vi "SpotFinder.vi"(0 "first scan?":bool, 1 "auto":bool, 4 "Int duplex?":refnum<vi>, 5 "notes":refnum<vi>, 6 "router 3":refnum<vi>, 7 "plane 2":refnum<vi>, 8 "Image Path":refnum<vi>, 9 "16bit?":refnum<vi>, 10 "TACwinLoaded?":refnum<vi>) -> ()   [LabVIEW 2009]
panel:
  out "already x spots":i16
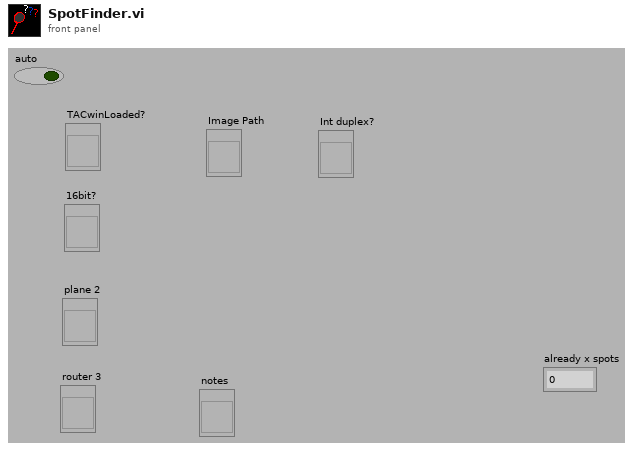
[diagram p1: front panel]
types:
  T1 = enum16{"Ini", "Dump", "Colorpal", "Input", "Get"}
  T2 = enum16{"Display", "change", "get", "save", "create text", "load", "Get Refnum"}
  T3 = enum16{"Ini", "Get", "Set", "Refresh", "dump", "move", "name"}
  T4 = typedef "spotproperties.ctl" = cluster{"draw?":bool, "plane":u32, "Coordinates":i32[], "TACWindow":cluster{"TACWindow1":i32, "TACWindow2":i32}, "Lifetime[ns]":ext[], "tauerror":dbl[], "F2-Value overall":dbl, "overall intensity":u32[], "F2-Value TAC":dbl, "TAC intensity":u32[], "Decay":u32[][]}
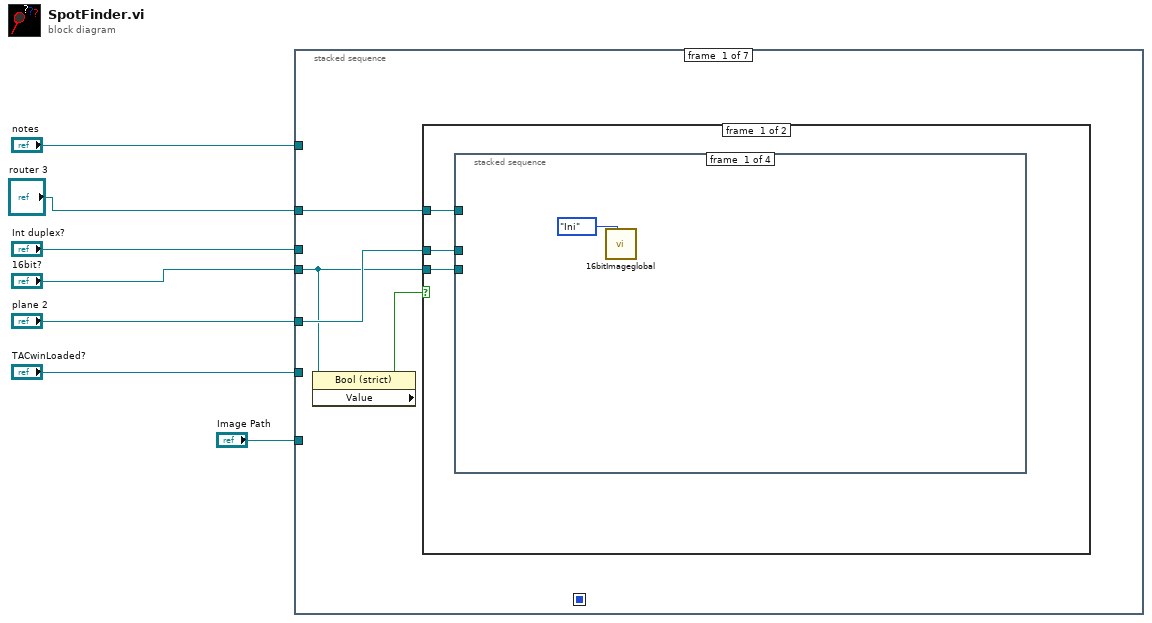
[diagram p0: block diagram]
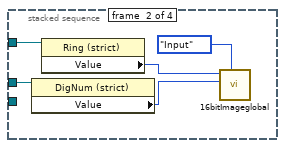
[diagram p2: hidden frame]
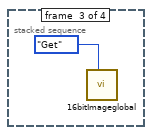
[diagram p3: hidden frame]
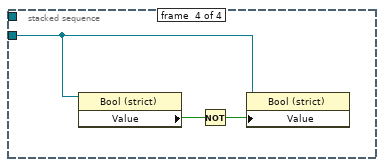
[diagram p4: hidden frame]
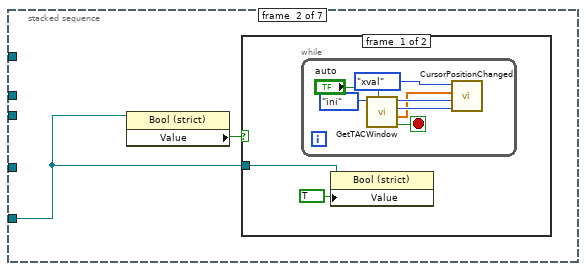
[diagram p6: hidden frame]
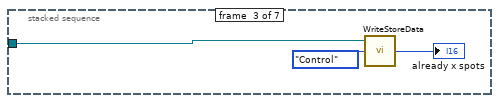
[diagram p8: hidden frame]
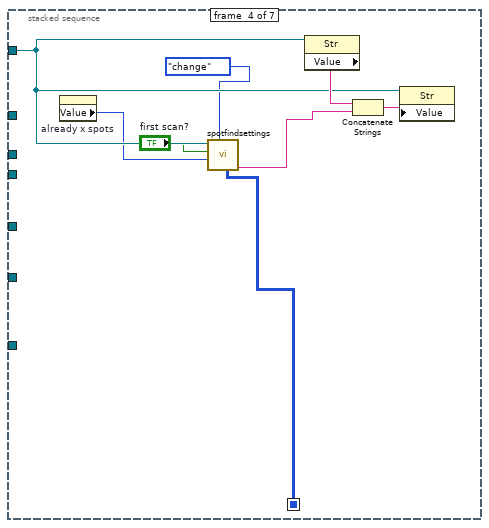
[diagram p9: hidden frame]
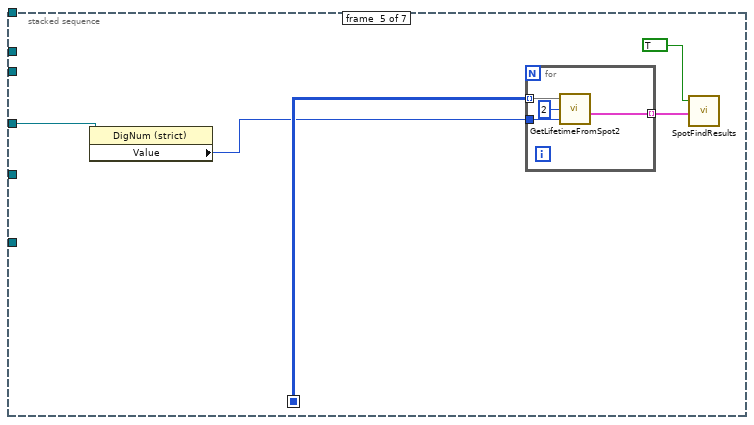
[diagram p10: hidden frame]
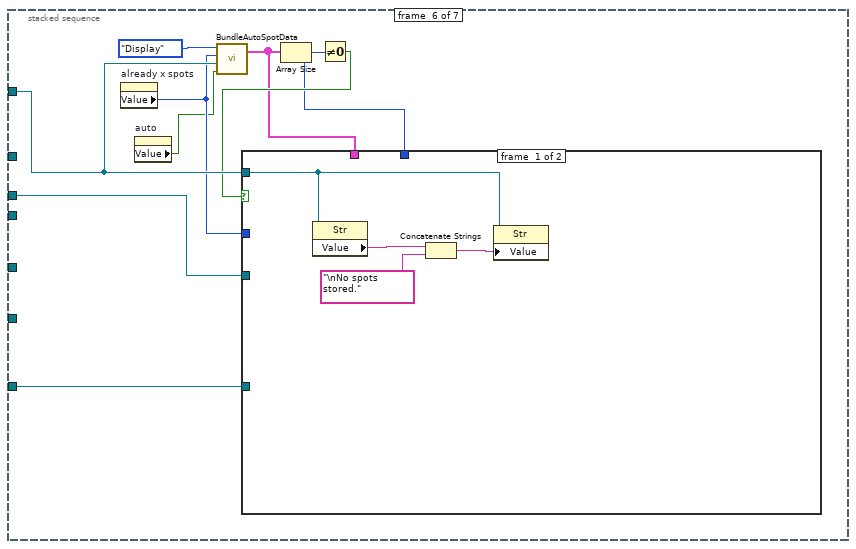
[diagram p11: hidden frame]
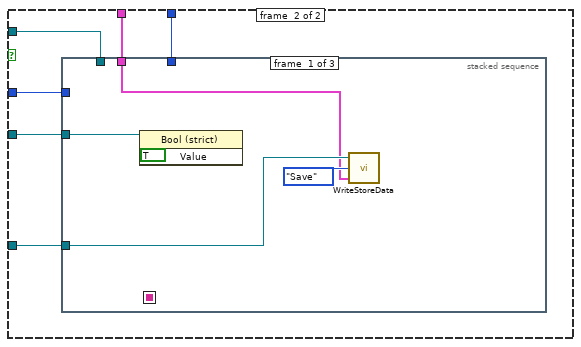
[diagram p12: hidden frame]
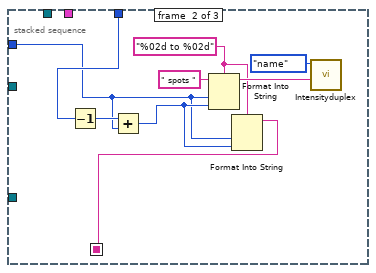
[diagram p13: hidden frame]
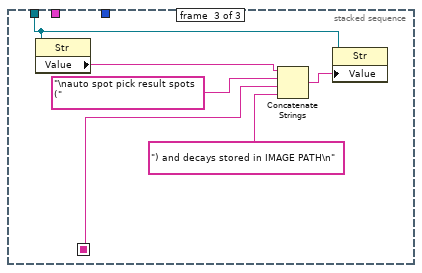
[diagram p14: hidden frame]
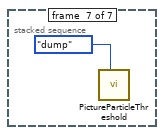
[diagram p15: hidden frame]
diagram:
  n1 = stacked-sequence {
    seq-local: [_ _ _ w40 _ _ _] -> [_ _ _ _ w51 _ _]
    tunnel: "TACwinLoaded?" -> [_ w25 _ _ _ _ _]
    tunnel: "router 3" -> [w10 _ _ _ _ _ _]
    tunnel: "plane 2" -> [w9 _ _ _ w50 _ _]
    tunnel: "16bit?" -> [w8 _ _ _ _ _ _]
    tunnel: "Int duplex?" -> [_ _ _ _ _ w64 _]
    tunnel: "notes" -> [_ _ _ w44 _ w62 _]
    tunnel: "Image Path" -> [_ _ w37 _ _ w63 _]
    frame #0 {
      n2 = property on="Property Node" class="Bool (strict)"(reference=w8) -> ("Value"=w11:bool)  [unwired: 1 in, 2 out]
      n3 = case shown="False" w11 {
        tunnel: w10 -> [w14 _]
        tunnel: w9 -> [w13 _]
        tunnel: w8 -> [w12 _]
        frame #0 {
          n4 = stacked-sequence {
            tunnel: w14 -> [_ w17 _ _]
            tunnel: w13 -> [_ w16 _ _]
            tunnel: w12 -> [_ _ _ w22]
            frame #0 {
              n5 = call "16bitImageglobal.vi"("Enum"=T1."Ini") -> ()  [unwired: 4 in, 4 out]
            }
            frame #1 {
              n6 = property on="Property Node" class="DigNum (strict)"(reference=w16) -> ("Value"=w19:u32)  [unwired: 1 in, 2 out]
              n7 = property on="Property Node" class="Ring (strict)"(reference=w17) -> ("Value"=w20:u8)  [unwired: 1 in, 2 out]
              n8 = call "16bitImageglobal.vi"("Enum"=T1."Input", "plane"=w19, "router"=w20) -> ()  [unwired: 2 in, 4 out]
            }
            frame #2 {
              n9 = call "16bitImageglobal.vi"("Enum"=T1."Get") -> ()  [unwired: 4 in, 4 out]
            }
            frame #3 {
              n10 = property on="Property Node" class="Bool (strict)"(reference=w22) -> ("Value"=w24:bool)  [unwired: 1 in, 2 out]
              n11 = Not(x=w24) -> (.not. x?=w23:bool)
              n12 = property on="Property Node" class="Bool (strict)"(reference=w22, "Value"=w23) -> ()  [unwired: 1 in, 2 out]
            }
          }
        }
        frame #1 {
        }
      }
    }
    frame #1 {
      n13 = property on="Property Node" class="Bool (strict)"(reference=w25) -> ("Value"=w26:bool)  [unwired: 1 in, 2 out]
      n14 = case shown="False" w26 {
        tunnel: w25 -> [w27 _]
        frame #0 {
          n15 = while {
            stop <- w34 stop-if-true
            n16 = call "GetTACWindow.vi"("Enum"=enum16{"ini", "get", "quick"}."ini", "auto"="auto") -> ("Cursor.Cursor Position:Cursor X"=w33:u16, "Cursor.Cursor Position:Cursor X 2"=w32:u16, "x-values"=w30:dbl[], "ready?"=w34:bool)  [unwired: 5 out]
            n17 = call "CursorPositionChanged.vi"("CursorPos x1"=w32, "CursorPos x0"=w33, "x-values"=w30, "action"=enum16{"Check", "Get", "xval"}."xval" ("Enum")) -> ()  [unwired: 4 out]
          }
          n18 = property on="Property Node" class="Bool (strict)"(reference=w27, "Value"=TRUE) -> ()  [unwired: 1 in, 2 out]
        }
        frame #1 {
        }
      }
    }
    frame #2 {
      n19 = call "WriteStoreData.vi"("Enum"=enum16{"Save", "Control"}."Control", "Image Path"=w37) -> ("already x spots"=→"already x spots":i16)  [unwired: 1 in]
    }
    frame #3 {
      n20 = property on="already x spots" class="Digital (strict)"() -> ("Value"=w43:i16)  [unwired: 2 in, 2 out]
      n21 = call "spotfindsettings.vi"("Enum"=T2."change", "already x spots found"=w43, "first scan?"="first scan?", "notes 2"=w44) -> ("settings"=w41:string, "coordinates"=w40:i32[][])  [unwired: 5 in, 1 out]
      n22 = property on="Property Node" class="Str"(reference=w44) -> ("Value"=w46:string)  [unwired: 1 in, 2 out]
      n23 = Concatenate Strings(w46, w41) -> (w45:string)
      n24 = property on="Property Node" class="Str"(reference=w44, "Value"=w45) -> ()  [unwired: 1 in, 2 out]
    }
    frame #4 {
      n25 = property class="DigNum (strict)"(reference=w50) -> ("Value"=w49:u32)  [unwired: 1 in, 2 out]
      n26 = for {
        tunnel: w51 -> [w55] mode=indexing
        tunnel: [w54] -> w47 mode=indexing
        tunnel: w49 -> [w53]
        n27 = call "GetLifetimeFromSpot2.vi"("plane"=w53, "F2-channel"=u8 2, "Coordinates"=w55) -> ("SpotProperties"=w54:T4)  [unwired: 5 in]
      }
      n28 = call "SpotFindResults.vi"("Spots in"=w47, "set?"=TRUE) -> ()  [unwired: 3 in, 1 out]
    }
    frame #5 {
      n29 = property on="already x spots" class="Digital (strict)"() -> ("Value"=w57:i16)  [unwired: 2 in, 2 out]
      n30 = property on="auto" class="Bool (strict)"() -> ("Value"=w56:bool)  [unwired: 2 in, 2 out]
      n31 = call "BundleAutoSpotData.vi"("auto"=w56, "notes 2"=w62, "already x spots"=w57, "Enum"=enum16{"1st sort", "Display", "Get"}."Display") -> ("Spots out"=w59:T4[])  [unwired: 1 in]
      n32 = Array Size(array=w59) -> (size(s)=w58:i32)
      n33 = Not Equal To 0?(x=w58) -> (x != 0?=w60:bool)
      n34 = case shown="True" w60 {
        tunnel: w59 -> [_ w74]
        tunnel: w58 -> [_ w73]
        tunnel: w64 -> [_ w72]
        tunnel: w62 -> [w65 w71]
        tunnel: w57 -> [_ w70]
        tunnel: w63 -> [_ w69]
        frame #0 {
          n35 = property on="Property Node" class="Str"(reference=w65) -> ("Value"=w68:string)  [unwired: 1 in, 2 out]
          n36 = Concatenate Strings(w68, "\nNo spots stored." ("string")) -> (w67:string)
          n37 = property on="Property Node" class="Str"(reference=w65, "Value"=w67) -> ()  [unwired: 1 in, 2 out]
        }
        frame #1 {
          n38 = stacked-sequence {
            seq-local: [_ w83 _] -> [_ _ w90]
            tunnel: w74 -> [w75 _ _]
            tunnel: w73 -> [_ w81 _]
            tunnel: w72 -> [w77 _ _]
            tunnel: w71 -> [_ _ w89]
            tunnel: w70 -> [_ w80 _]
            tunnel: w69 -> [w76 _ _]
            frame #0 {
              n39 = property on="Property Node" class="Bool (strict)"(reference=w77, "Value"=TRUE ("Boolean 2")) -> ()  [unwired: 1 in, 2 out]
              n40 = call "WriteStoreData.vi"("Spots"=w75, "Enum"=enum16{"Save", "Control"}."Save", "Image Path"=w76) -> ()  [unwired: 1 out]
            }
            frame #1 {
              w85 = "%02d to %02d" ("format string")
              n41 = Decrement(x=w81) -> (x-1=w84:i32)
              n42 = Add(x=w84, y=w80) -> (x+y=w82:i32)
              n43 = Format Into String(format string=w85, initial string=" spots ", w80, w82) -> (resulting string=w86:string)  [unwired: 1 in, 1 out]
              n44 = Format Into String(format string=w85, w80, w82) -> (resulting string=w83:string)  [unwired: 2 in, 1 out]
              n45 = call "Intensityduplex.vi"("Enum"=T3."name", "add string"=w86) -> ()  [unwired: 3 in, 2 out]
            }
            frame #2 {
              n46 = property on="Property Node" class="Str"(reference=w89) -> ("Value"=w93:string)  [unwired: 1 in, 2 out]
              n47 = Concatenate Strings(w93, "\nauto spot pick result spots (" ("string"), w90, ") and decays stored in IMAGE PATH\n" ("string")) -> (w92:string)
              n48 = property on="Property Node" class="Str"(reference=w89, "Value"=w92) -> ()  [unwired: 1 in, 2 out]
            }
          }
        }
      }
    }
    frame #6 {
      n49 = call "PictureParticleThreshold.vi"("Enum"=enum16{"new", "input", "draw", "dump"}."dump") -> ()  [unwired: 7 in, 2 out]
    }
  }
